vi "Subset_Array.vi"(0 "Subset Array 1D":i8[](array[numeric])=[0, 1, 2, 3, 4], 1 "Index Subset":i32, 2 "Length Subset":i32, 3 "Subset Array 2D":i8[][](array[numeric])=[[-5, -1, 3], [-4, 0, 4], [-3, 1, 5], [-2, 2, 6]], 4 "Indexs SA":T2={"Rows"=-1, "Columns"=-1} {"Columns" min=-1; "Rows" min=-1}, 5 "Lengths R&C":T1, 8 "Choose Subset Array":T3) -> (15 "SubArray 1D":i8[](array[numeric]), 18 "SubArray 2D":i8[][](array[numeric]))   [LabVIEW 2018]
uses:
  Controls/1D_2D.ctl
  Controls/Rows_Columns.ctl
  Controls/Lengths_Rows_Columns.ctl
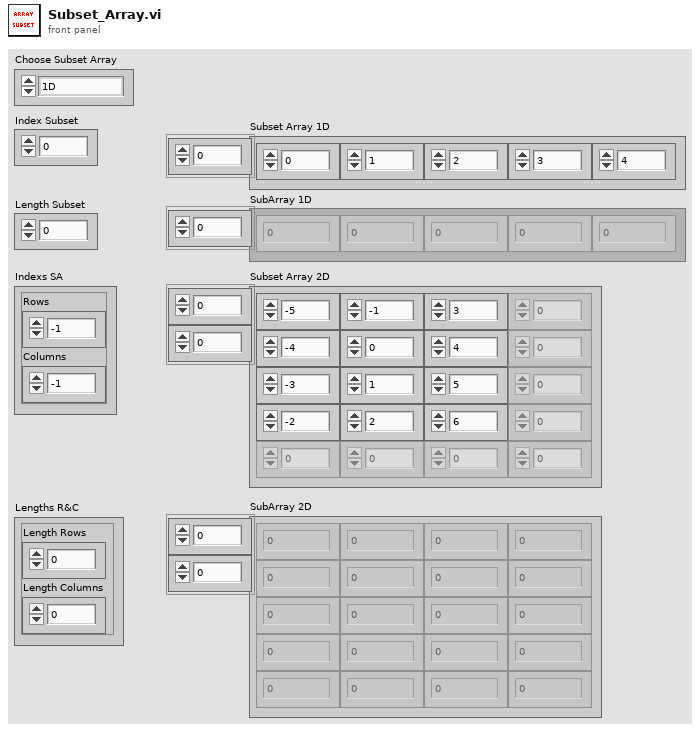
[diagram p1: front panel]
types:
  T1 = typedef "Lengths_Rows_Columns.ctl" = cluster{"Length Rows":i32, "Length Columns":i32}
  T2 = typedef "Rows_Columns.ctl" = cluster{"Rows":i32, "Columns":i32}
  T3 = typedef "1D_2D.ctl" = enum16{"1D", "2D"}
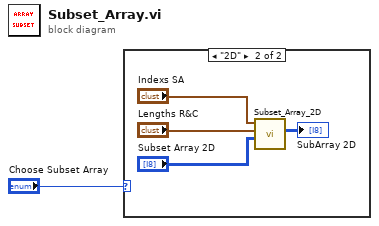
[diagram p0: block diagram]
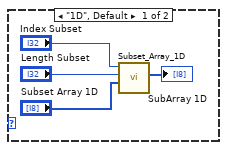
[diagram p2: hidden frame]
diagram:
  n1 = case shown="\"2D\"" "Choose Subset Array" {
    frame "1D", Default {
      n2 = call "Subset_Array_1D.vi"("Subset Array 1D"="Subset Array 1D", "Length Subset"="Length Subset", "Index Subset"="Index Subset") -> ("SubArray 1D"=→"SubArray 1D":i8[])  [unwired: 8 in]
    }
    frame "2D" {
      n3 = call "Subset_Array_2D.vi"("Subset Array 2D"="Subset Array 2D", "Lengths R&C"="Lengths R&C", "Indexs SA"="Indexs SA") -> ("SubArray 2D"=→"SubArray 2D":i8[][])  [unwired: 8 in]
    }
  }
